vi "Symphony Format CrvNames.vi"(5 "Noise Mode":T1=enum."Selected Curve", 6 "NoiseWindow":bool, 7 "error in (no error)":errorcluster, 9 "Accumulation":i32=1 min=1 max=256 step=1, 10 "numAreas":i32=1) -> (0 "error out":errorcluster, 1 "DatDisplayNm":string[](array[string]), 2 "VarParY":dbl[](array[numeric]), 3 "SubDatDisplayNm":string[](array[string]))   [LabVIEW 2019]
uses:
  <userlib>/JY Symphony/NoiseCorr.ctl
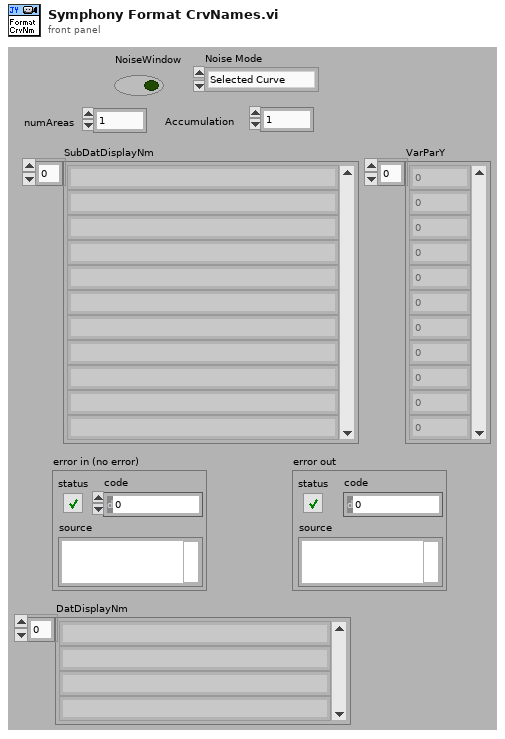
[diagram p1: front panel]
types:
  T1 = typedef "NoiseCorr.ctl" = enum16{"Off", "Selected Curve", "One For Every Acq"}
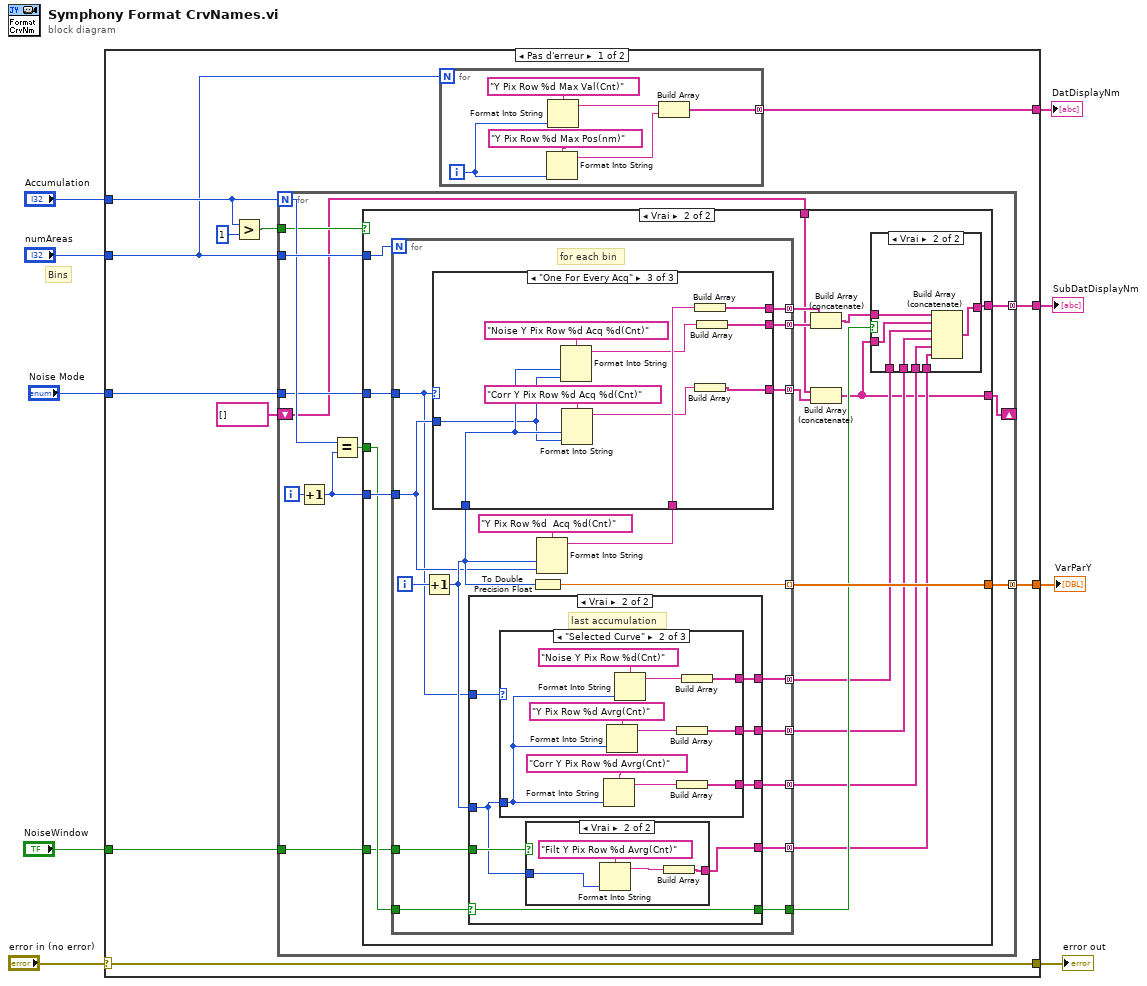
[diagram p0: block diagram]
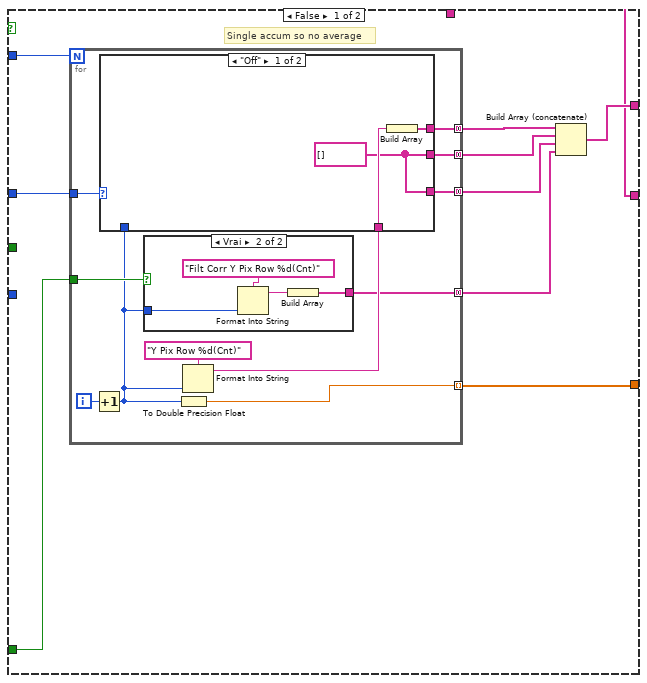
[diagram p2: hidden frame]
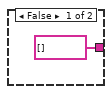
[diagram p3: hidden frame]
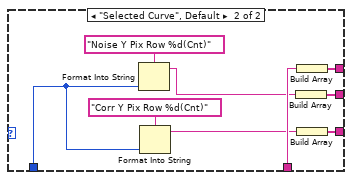
[diagram p4: hidden frame]
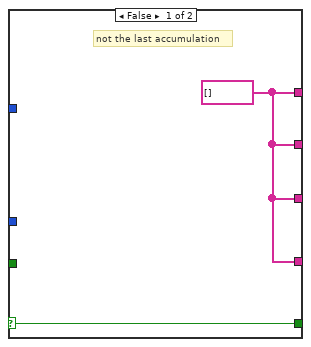
[diagram p6: hidden frame]
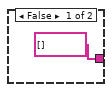
[diagram p7: hidden frame]
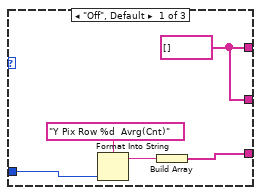
[diagram p8: hidden frame]
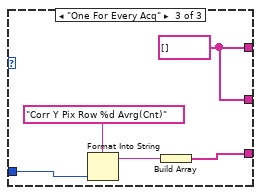
[diagram p9: hidden frame]
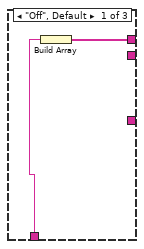
[diagram p10: hidden frame]
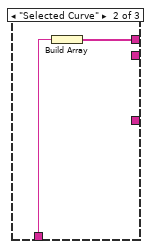
[diagram p11: hidden frame]
diagram:
  # "Bins"
  n1 = case shown="Pas d'erreur" "error in (no error)" {
    selector: "error in (no error)" -> [w18 w169]
    tunnel: "numAreas" -> [w11 _]
    tunnel: "Accumulation" -> [w17 _]
    tunnel: [w18 w169] -> w6
    tunnel: [w20 _] -> w5
    tunnel: [w19 _] -> w4
    tunnel: "NoiseWindow" -> [w14 _]
    tunnel: "Noise Mode" -> [w13 _]
    tunnel: [w10 _] -> w1
    frame No Error {
      n2 = Greater?(x=w17, y=1) -> (0:w15:bool)
      n3 = for {
        N: w17 -> [w27]
        tunnel: [w32] -> w20 mode=concatenating
        tunnel: [w31] -> w19 mode=concatenating
        tunnel: w11 -> [w30]
        tunnel: w15 -> [w23]
        tunnel: w14 -> [w25]
        tunnel: w13 -> [w24]
        shift-right: [w22] -> _
        shift-left: string[] [] -> [w21]
        i -> [w29]
        n4 = Increment(x=w29) -> (x+1=w28:i32)
        n5 = Equal?(x=w27, y=w28) -> (x = y?=w26:bool)
        n6 = case shown="Vrai" w23 {
          tunnel: [w37 w83] -> w32
          tunnel: [w41 w88] -> w31
          tunnel: w30 -> [w40 w87]
          tunnel: w28 -> [_ w86]
          tunnel: w26 -> [_ w85]
          tunnel: w25 -> [w39 w81]
          tunnel: w24 -> [w38 w80]
          tunnel: [w33 w71] -> w22
          tunnel: w21 -> [w33 w73]
          frame False {
            # "Single accum so no average"
            n7 = for {
              N: w40 -> [_]
              tunnel: [w53] -> w41 mode=indexing
              tunnel: [w49] -> w42 mode=concatenating
              tunnel: w39 -> [w45]
              tunnel: w38 -> [w48]
              tunnel: [w47] -> w36 mode=concatenating
              tunnel: [w46] -> w35 mode=concatenating
              tunnel: [w43] -> w34 mode=concatenating
              i -> [w52]
              n8 = Increment(x=w52) -> (x+1=w44:i32)
              n9 = case shown="Vrai" w45 {
                tunnel: w44 -> [_ w57]
                tunnel: [string[] [] w55] -> w43
                frame False {
                }
                frame True {
                  n10 = Format Into String(format string="Filt Corr Y Pix Row %d(Cnt)", w57) -> (resulting string=w56:string)  [unwired: 2 in, 1 out]
                  n11 = Build Array(w56) -> (w55:string[])
                }
              }
              n12 = To Double Precision Float(number=w44) -> (double precision float=w53:dbl)
              n13 = Format Into String(format string="Y Pix Row %d(Cnt)", w44) -> (resulting string=w50:string)  [unwired: 2 in, 1 out]
              n14 = case shown="\"Off\"" w48 {
                tunnel: w50 -> [w61 w69]
                tunnel: [w60 w70] -> w49
                tunnel: w44 -> [_ w68]
                tunnel: [w59 w67] -> w47
                tunnel: [w59 w66] -> w46
                frame "Off" {
                  w59 = string[] []
                  n15 = Build Array(w61) -> (w60:string[])
                }
                frame "Selected Curve", Default {
                  n16 = Format Into String(format string="Noise Y Pix Row %d(Cnt)", w68) -> (resulting string=w62:string)  [unwired: 2 in, 1 out]
                  n17 = Format Into String(format string="Corr Y Pix Row %d(Cnt)", w68) -> (resulting string=w63:string)  [unwired: 2 in, 1 out]
                  n18 = Build Array(w62) -> (w66:string[])
                  n19 = Build Array(w69) -> (w70:string[])
                  n20 = Build Array(w63) -> (w67:string[])
                }
              }
            }
            n21 = Build Array (concatenate)(w42, w35, w36, w34) -> (w37:string[])
          }
          frame True {
            n22 = for {
              N: w87 -> [_]
              tunnel: [w113] -> w88 mode=indexing
              tunnel: [w110] -> w76 mode=concatenating
              tunnel: w86 -> [w104]
              tunnel: w85 -> [w108]
              tunnel: [w106] -> w82 mode=concatenating
              tunnel: [w105] -> w84
              tunnel: w81 -> [w102]
              tunnel: w80 -> [w103]
              tunnel: [w101] -> w77 mode=concatenating
              tunnel: [w100] -> w78 mode=concatenating
              tunnel: [w99] -> w79 mode=concatenating
              tunnel: [w98] -> w72 mode=concatenating
              tunnel: [w97] -> w75 mode=concatenating
              i -> [w109]
              # "for each bin"
              n23 = Increment(x=w109) -> (x+1=w107:i32)
              n24 = case shown="Vrai" w108 {
                selector: w108 -> [w115 w123]
                tunnel: w107 -> [_ w117]
                tunnel: [w114 w116] -> w106
                tunnel: [w115 w123] -> w105
                tunnel: w103 -> [_ w122]
                tunnel: w102 -> [_ w118]
                tunnel: [w114 w121] -> w101
                tunnel: [w114 w120] -> w100
                tunnel: [w114 w119] -> w99
                frame False {
                  w114 = string[] []
                  # "not the last accumulation"
                }
                frame True {
                  # "last accumulation"
                  n25 = case shown="\"Selected Curve\"" w122 {
                    tunnel: w117 -> [w131 w143 w148]
                    tunnel: [w129 w138 w146] -> w121
                    tunnel: [w129 w136 w146] -> w120
                    tunnel: [w130 w134 w144] -> w119
                    frame "Off", Default {
                      w129 = string[] []
                      n26 = Format Into String(format string="Y Pix Row %d  Avrg(Cnt)", w131) -> (resulting string=w133:string)  [unwired: 2 in, 1 out]
                      n27 = Build Array(w133) -> (w130:string[])
                    }
                    frame "Selected Curve" {
                      n28 = Format Into String(format string="Corr Y Pix Row %d Avrg(Cnt)", w143) -> (resulting string=w135:string)  [unwired: 2 in, 1 out]
                      n29 = Format Into String(format string="Y Pix Row %d Avrg(Cnt)", w143) -> (resulting string=w137:string)  [unwired: 2 in, 1 out]
                      n30 = Format Into String(format string="Noise Y Pix Row %d(Cnt)", w143) -> (resulting string=w139:string)  [unwired: 2 in, 1 out]
                      n31 = Build Array(w137) -> (w136:string[])
                      n32 = Build Array(w135) -> (w134:string[])
                      n33 = Build Array(w139) -> (w138:string[])
                    }
                    frame "One For Every Acq" {
                      w146 = string[] []
                      n34 = Format Into String(format string="Corr Y Pix Row %d Avrg(Cnt)", w148) -> (resulting string=w147:string)  [unwired: 2 in, 1 out]
                      n35 = Build Array(w147) -> (w144:string[])
                    }
                  }
                  n36 = case shown="Vrai" w118 {
                    tunnel: w117 -> [_ w128]
                    tunnel: [string[] [] w127] -> w116
                    frame False {
                    }
                    frame True {
                      n37 = Format Into String(format string="Filt Y Pix Row %d Avrg(Cnt)", w128) -> (resulting string=w126:string)  [unwired: 2 in, 1 out]
                      n38 = Build Array(w126) -> (w127:string[])
                    }
                  }
                }
              }
              n39 = To Double Precision Float(number=w107) -> (double precision float=w113:dbl)
              n40 = Format Into String(format string="Y Pix Row %d  Acq %d(Cnt)", w107, w104) -> (resulting string=w111:string)  [unwired: 2 in, 1 out]
              n41 = case shown="\"One For Every Acq\"" w103 {
                tunnel: w111 -> [w150 w151 w162]
                tunnel: [w149 w152 w158] -> w110
                tunnel: w107 -> [_ _ w161]
                tunnel: w104 -> [_ _ w153]
                tunnel: [_ _ w160] -> w98
                tunnel: [_ _ w159] -> w97
                frame "Off", Default {
                  n42 = Build Array(w150) -> (w149:string[])
                }
                frame "Selected Curve" {
                  n43 = Build Array(w151) -> (w152:string[])
                }
                frame "One For Every Acq" {
                  n44 = Format Into String(format string="Noise Y Pix Row %d Acq %d(Cnt)", w161, w153) -> (resulting string=w154:string)  [unwired: 2 in, 1 out]
                  n45 = Format Into String(format string="Corr Y Pix Row %d Acq %d(Cnt)", w161, w153) -> (resulting string=w155:string)  [unwired: 2 in, 1 out]
                  n46 = Build Array(w162) -> (w158:string[])
                  n47 = Build Array(w155) -> (w160:string[])
                  n48 = Build Array(w154) -> (w159:string[])
                }
              }
            }
            n49 = Build Array (concatenate)(w76, w75) -> (w74:string[])
            n50 = Build Array (concatenate)(w73, w72) -> (w71:string[])
            n51 = case shown="Vrai" w84 {
              tunnel: w74 -> [w89 w95]
              tunnel: [w89 w96] -> w83
              tunnel: w82 -> [_ w94]
              tunnel: w79 -> [_ w93]
              tunnel: w78 -> [_ w92]
              tunnel: w77 -> [_ w91]
              tunnel: w71 -> [_ w90]
              frame False {
              }
              frame True {
                n52 = Build Array (concatenate)(w95, w90, w91, w92, w93, w94) -> (w96:string[])
              }
            }
          }
        }
      }
      n53 = for {
        N: w11 -> [_]
        tunnel: [w164] -> w10 mode=concatenating
        i -> [w163]
        n54 = Format Into String(format string="Y Pix Row %d Max Pos(nm)", w163) -> (resulting string=w165:string)  [unwired: 2 in, 1 out]
        n55 = Format Into String(format string="Y Pix Row %d Max Val(Cnt)", w163) -> (resulting string=w166:string)  [unwired: 2 in, 1 out]
        n56 = Build Array(w166, w165) -> (w164:string[])
      }
    }
    frame Error {
    }
  }
  "error out" <- w6
  "SubDatDisplayNm" <- w5
  "VarParY" <- w4
  "DatDisplayNm" <- w1
